vi "Server Side.vi"() -> ()   [LabVIEW 2021]
uses:
  <vilib>/Utility/file.llb/Write Delimited Spreadsheet (string).vi
panel:
  out "Server Error":errorcluster
  out "SERVICE TYPE":string
  out "TIME":string
  out "DATE":string
  # "SERVER LOG"
  # "ERROR HANDLING"
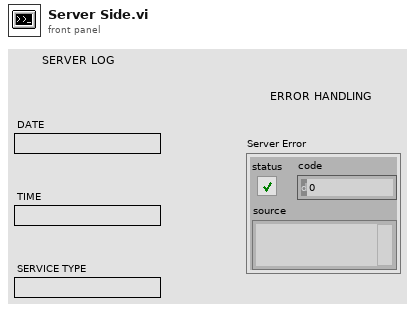
[diagram p1: front panel]
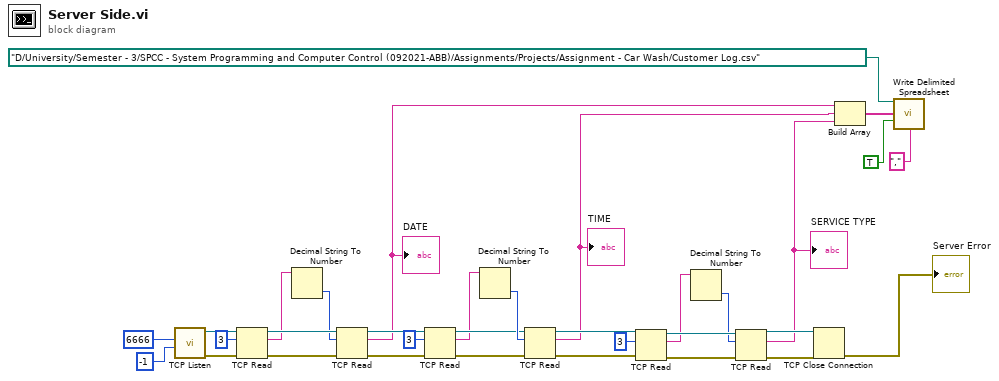
[diagram p0: block diagram]
diagram:
  n1 = call <vilib>:"TCP Listen.vi"("timeout ms (wait forever: -1)"=-1, "port"=u16 6666) -> ("error out"=w29:errorcluster, "connection ID"=w31:refnum<k5>)  [unwired: 5 in, 3 out]
  n2 = TCP Read(connection ID=w31, bytes to read=3, error in (no error)=w29) -> (connection ID out=w30:refnum<k5>, data out=w27:string, error out=w28:errorcluster)  [unwired: 2 in]
  n3 = Decimal String To Number(string=w27) -> (number=w26:i32)  [unwired: 2 in, 1 out]
  n4 = TCP Read(connection ID=w30, bytes to read=w26, error in (no error)=w28) -> (connection ID out=w13:refnum<k5>, data out=w8:string, error out=w16:errorcluster)  [unwired: 2 in]
  "DATE" <- w8
  n5 = TCP Read(connection ID=w13, bytes to read=3, error in (no error)=w16) -> (connection ID out=w21:refnum<k5>, data out=w7:string, error out=w22:errorcluster)  [unwired: 2 in]
  n6 = Decimal String To Number(string=w7) -> (number=w23:i32)  [unwired: 2 in, 1 out]
  n7 = TCP Read(connection ID=w21, bytes to read=w23, error in (no error)=w22) -> (connection ID out=w12:refnum<k5>, data out=w5:string, error out=w15:errorcluster)  [unwired: 2 in]
  "TIME" <- w5
  n8 = TCP Read(connection ID=w12, bytes to read=3, error in (no error)=w15) -> (connection ID out=w20:refnum<k5>, data out=w18:string, error out=w19:errorcluster)  [unwired: 2 in]
  n9 = Decimal String To Number(string=w18) -> (number=w17:i32)  [unwired: 2 in, 1 out]
  n10 = TCP Read(connection ID=w20, bytes to read=w17, error in (no error)=w19) -> (connection ID out=w11:refnum<k5>, data out=w6:string, error out=w14:errorcluster)  [unwired: 2 in]
  "SERVICE TYPE" <- w6
  n11 = TCP Close Connection(connection ID=w11, error in (no error)=w14) -> (error out=→"Server Error":errorcluster)  [unwired: 1 in, 1 out]
  n12 = Build Array(w8, w5, w6) -> (w4:string[])
  n13 = call-poly <vilib>:"Write Delimited Spreadsheet.vi"("file path (dialog if empty)"=path "D:/University/Semester - 3/SPCC - System Programming and Computer Control (092021-ABB)/Assignments/Projects/Assignment - Car Wash/Customer Log.csv", "1D data"=w4, "append to file? (new file:F)"=TRUE, "delimiter (\\t)"="," ("delimiter (\\t)")) -> ()  [unwired: 10 in, 2 out]
